vi "Configure.vi"(8 "error in (no error)":errorcluster) -> (0 "error out":errorcluster, 3 "name":string)   [LabVIEW 2013]
uses:
  INI/INIstring.vi
  SubVi/Global constant.vi
  INI/INIi32.vi
  INI/INIpath.vi
  <vilib>/Utility/config.llb/NI_LVConfig.lvlib
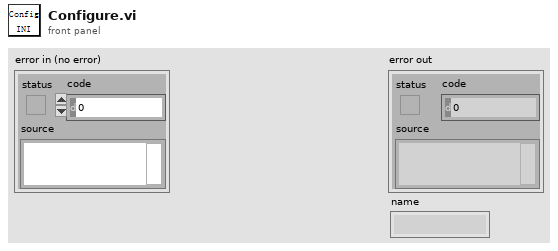
[diagram p1: front panel]
types:
  T1 = typedef "NI_LVConfig.lvlib/Config Data RefNum.ctl" = refnum<k1>
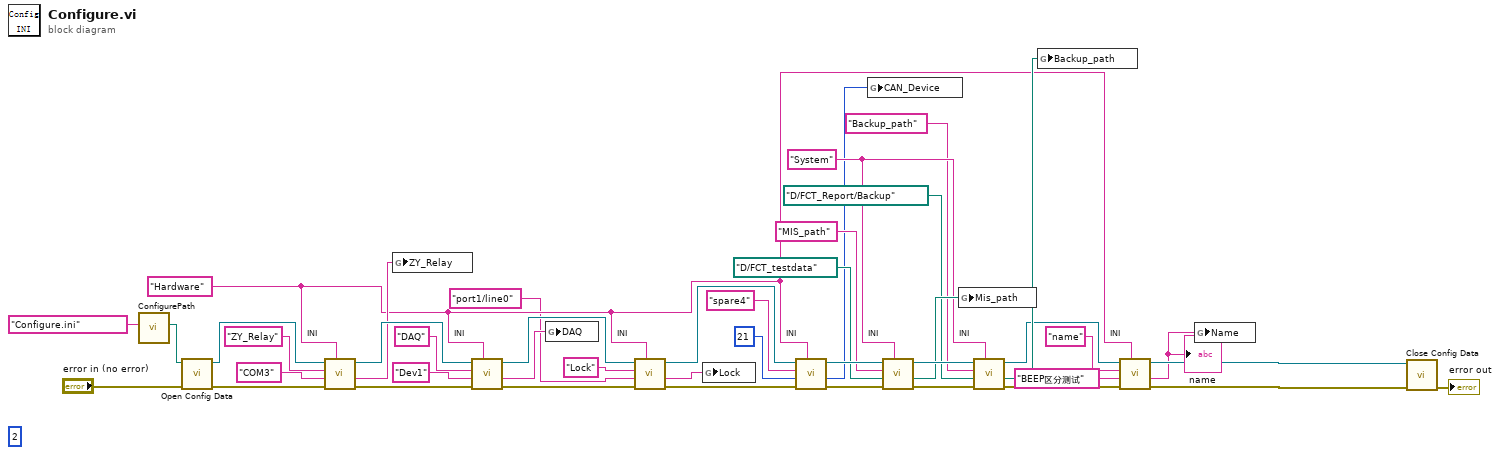
[diagram p0: block diagram]
diagram:
  w14 = "System" ("Section")
  (unwired) 2 ("default value")
  w5 = "Hardware" ("Section")
  n1 = call "ConfigurePath.vi"("ConfigureName"="Configure.ini") -> ("Filepath"=w32:path)  [unwired: 7 in, 3 out]
  n2 = call <vilib>:"Open Config Data.vi"("error in (no error)"="error in (no error)", "configuration file path"=w32) -> ("error out"=w34:errorcluster, "refnum"=w36:T1)  [unwired: 7 in, 1 out]
  n3 = call-poly "INI.vi"("Section"=w5, "error in (no error)"=w34, "default value"="COM3", "Key"="ZY_Relay", "Refnum in"=w36) -> ("Error Out"=w33:errorcluster, "Value"=w21:string, "Refnum out"=w35:T1)  [unwired: 4 in]
  n4 = global write "Global constant.vi" "ZY_Relay"(w21) -> ()
  n5 = call-poly "INI.vi"("Section"=w5, "error in (no error)"=w33, "default value"="Dev1", "Key"="DAQ", "Refnum in"=w35) -> ("Error Out"=w40:errorcluster, "Value"=w23:string, "Refnum out"=w42:T1)  [unwired: 4 in]
  n6 = global write "Global constant.vi" "DAQ"(w23) -> ()
  n7 = call-poly "INI.vi"("Section"=w5, "error in (no error)"=w40, "default value"="port1/line0", "Key"="Lock", "Refnum in"=w42) -> ("Error Out"=w39:errorcluster, "Value"=w22:string, "Refnum out"=w41:T1)  [unwired: 4 in]
  n8 = global write "Global constant.vi" "Lock"(w22) -> ()
  n9 = call-poly "INI.vi"("Section"=w5, "error in (no error)"=w39, "default value"=21, "Key"="spare4", "Refnum in"=w41) -> ("Error Out"=w37:errorcluster, "Value"=w11:i32, "Refnum out"=w38:T1)  [unwired: 4 in]
  n10 = global write "Global constant.vi" "CAN_Device"(w11) -> ()
  n11 = call-poly "INI.vi"("Section"=w14, "error in (no error)"=w37, "default value"=path "D:/FCT_testdata", "Key"="MIS_path", "Refnum in"=w38) -> ("Error Out"=w17:errorcluster, "Value"=w16:path, "Refnum out"=w18:T1)  [unwired: 4 in]
  n12 = global write "Global constant.vi" "Mis_path"(w16) -> ()
  n13 = call-poly "INI.vi"("Section"=w14, "error in (no error)"=w17, "default value"=path "D:/FCT_Report/Backup", "Key"="Backup_path", "Refnum in"=w18) -> ("Error Out"=w8:errorcluster, "Value"=w15:path, "Refnum out"=w10:T1)  [unwired: 4 in]
  n14 = global write "Global constant.vi" "Backup_path"(w15) -> ()
  n15 = call-poly "INI.vi"("Section"=w5, "error in (no error)"=w8, "default value"="BEEP区分测试", "Key"="name", "Refnum in"=w10) -> ("Error Out"=w7:errorcluster, "Value"=w6:string, "Refnum out"=w9:T1)  [unwired: 4 in]
  "name" <- w6
  n16 = global write "Global constant.vi" "Name"(w6) -> ()
  n17 = call <vilib>:"Close Config Data.vi"("error in (no error)"=w7, "refnum"=w9) -> ("error out"=→"error out":errorcluster)  [unwired: 8 in, 1 out]
